vi "Data Processing.vi"(5 "V to uS Conversion":dbl, 6 "uS Low":dbl, 7 "Samples Per Average":i32, 8 "Time":dbl, 9 "Conductivity Array":dbl[](array[numeric]), 10 "Thermocouple 2 Array":dbl[](array[numeric]), 11 "Data in":dbl[][](array[numeric])) -> (0 "Most Recent T2":dbl, 1 "Thermocouple Graph":cluster{"X":dbl, "Y":dbl}[](array[cluster]), 2 "Conductivity Meter Graph":cluster{"X":dbl, "Y":dbl}[](array[cluster]), 3 "Data out":dbl[][](array[numeric]), 4 "uS Array Out":dbl[](array[numeric]))   [LabVIEW 2016]
panel:
  out "Most Recent Conductivity":dbl
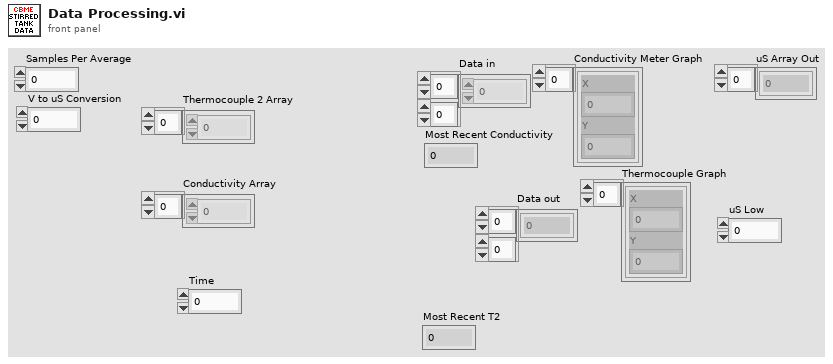
[diagram p1: front panel]
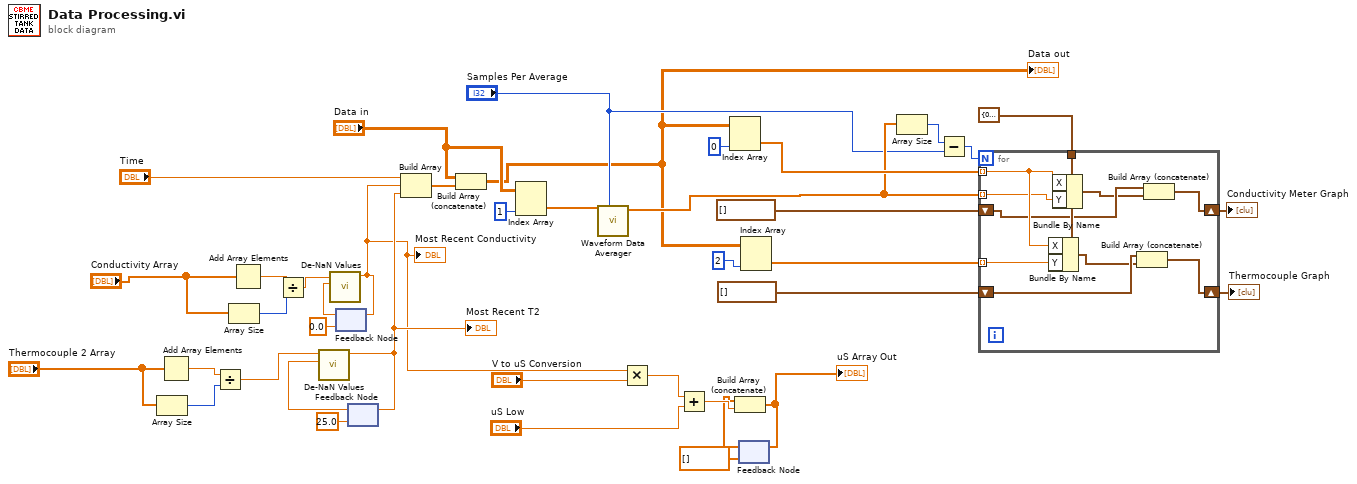
[diagram p0: block diagram]
diagram:
  n1 = Array Size(array="Thermocouple 2 Array") -> (size(s)=w38:i32)
  n2 = Add Array Elements(numeric array="Thermocouple 2 Array") -> (sum=w39:dbl)
  n3 = Divide(x=w39, y=w38) -> (x/y=w32:dbl)
  n4 = Array Size(array="Conductivity Array") -> (size(s)=w37:i32)
  n5 = Add Array Elements(numeric array="Conductivity Array") -> (sum=w36:dbl)
  n6 = Divide(x=w36, y=w37) -> (x/y=w28:dbl)
  n7 = feedback #1(0.0 ("De-NaN")) -> (w27:dbl)
  n8 = call "De-NaN Values.vi"("Last Valid"=w27, "Input"=w28) -> ("De-NaN"=w8:dbl)  [unwired: 9 in]
  "Most Recent Conductivity" <- w8
  n9 = feedback-in #1(w8) -> ()
  n10 = feedback #2(25.0 ("De-NaN")) -> (w31:dbl)
  n11 = call "De-NaN Values.vi"("Last Valid"=w31, "Input"=w32) -> ("De-NaN"=w29:dbl)  [unwired: 9 in]
  "Most Recent T2" <- w29
  n12 = feedback-in #2(w29) -> ()
  n13 = Build Array("Time", w8, w29) -> (w34:dbl[])
  n14 = Build Array (concatenate)("Data in", w34) -> (w9:dbl[][])
  "Data out" <- w9
  n15 = Index Array(array="Data in", index (col)=1 ("disabled index (col)")) -> (element=w25:dbl[])  [unwired: 1 in]
  n16 = call "Waveform Data Averager.vi"("Samples Per Average"="Samples Per Average", "Voltage Array In"=w25) -> ("Voltage Array Out"=w14:dbl[])  [unwired: 8 in, 1 out]
  n17 = Multiply(x=w8, y="V to uS Conversion") -> (x*y=w6:dbl)
  n18 = Add(x=w6, y="uS Low") -> (x+y=w4:dbl)
  n19 = Index Array(array=w9, index (col)=0 ("disabled index (col)")) -> (element=w16:dbl[])  [unwired: 1 in]
  n20 = feedback #3(dbl[] []) -> (w3:dbl[])
  n21 = Build Array (concatenate)(w3, w4) -> (w2:dbl[])
  "uS Array Out" <- w2
  n22 = feedback-in #3(w2) -> ()
  n23 = Index Array(array=w9, index (col)=2 ("disabled index (col)")) -> (element=w15:dbl[])  [unwired: 1 in]
  n24 = Array Size(array=w14) -> (size(s)=w13:i32)
  n25 = Subtract(x=w13, y="Samples Per Average") -> (x-y=w12:i32)
  n26 = for {
    N: w12 -> [_]
    shift-right: [w42] -> w18
    shift-left: cluster{"X":dbl, "Y":dbl}[] [] ("Conductivity Meter Graph") -> [w47]
    shift-right: [w43] -> w17
    shift-left: cluster{"X":dbl, "Y":dbl}[] [] ("Conductivity Meter Graph") -> [w45]
    tunnel: cluster{"X":dbl, "Y":dbl} {"X"=0.0, "Y"=0.0} -> [w50]
    tunnel: w16 -> [w49] mode=indexing
    tunnel: w15 -> [w48] mode=indexing
    tunnel: w14 -> [w41] mode=indexing
    n27 = Bundle By Name(cluster=w50, "X"=w49, "Y"=w48) -> (w44:cluster{"X":dbl, "Y":dbl})
    n28 = Bundle By Name(cluster=w50, "X"=w49, "Y"=w41) -> (w46:cluster{"X":dbl, "Y":dbl})
    n29 = Build Array (concatenate)(w45, w44) -> (w43:cluster{"X":dbl, "Y":dbl}[])
    n30 = Build Array (concatenate)(w47, w46) -> (w42:cluster{"X":dbl, "Y":dbl}[])
  }
  "Conductivity Meter Graph" <- w18
  "Thermocouple Graph" <- w17
